vi "Hydrostat.vi"() -> ()   [LabVIEW 2016]
uses:
  <vilib>/express/express signal manip/GetorSetDDTAttributes/Shared VIs/TimeType.ctl
  <vilib>/Waveform/WDTOps.llb/WDT Append Waveforms DBL.vi
  <vilib>/express/express signal manip/GetorSetDDTAttributes/Shared VIs/TimeMode Enum to Boolean.vi
  <vilib>/express/express shared/transition.llb/Dynamic To Waveform Array.vi
  <vilib>/express/express signal manip/GetorSetDDTAttributes/Set DDT Attributes/SetT0.vi
  <vilib>/express/express signal manip/GetorSetDDTAttributes/Set DDT Attributes/sub Set StartTimeStamp.vi
  <vilib>/express/express shared/transition.llb/Waveform Array To Dynamic.vi
  <vilib>/express/express signal manip/GetorSetDDTAttributes/Set DDT Attributes/Set DDT Properties.xnode
  <vilib>/express/express signal manip/GetorSetDDTAttributes/Shared VIs/GetSetShared.lvlib
  <vilib>/express/express signal manip/GetorSetDDTAttributes/Set DDT Attributes/Set DDT Attributes.lvlib
panel:
  in  "Test Name":string caption="Comment"
  in  "Stop Button":bool
  out "Waveform Chart":waveform(dbl)(graph)
  out "PSIA":dbl format="%.2f"
  in  "Outlet":bool
  in  "Mix 2":bool
  in  "Mix 1":bool
  in  "Grease":bool
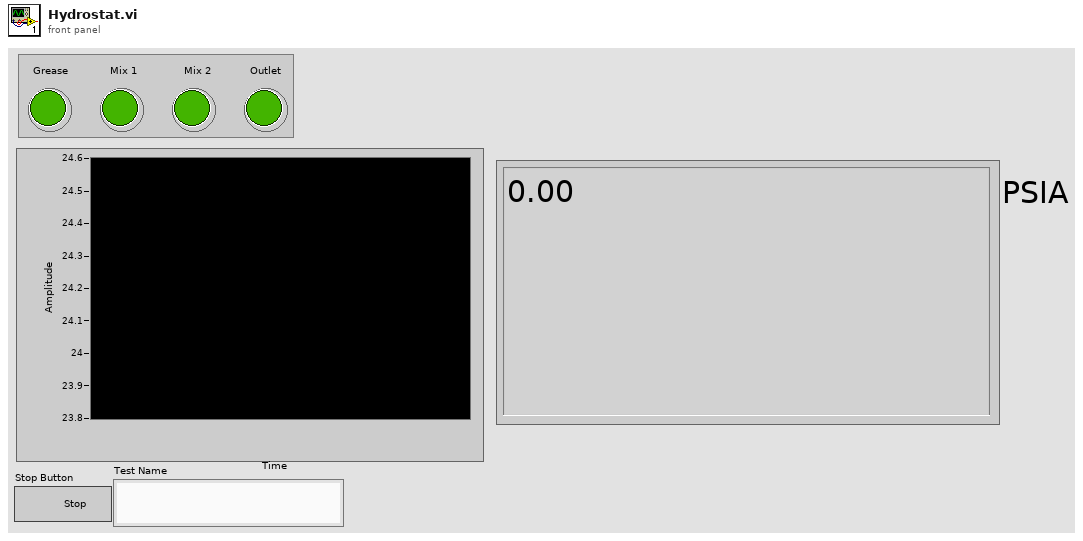
[diagram p1: front panel]
types:
  T1 = typedef "GetSetShared.lvlib/TimeType.ctl" = enum16{"Absolute", "Relative"}
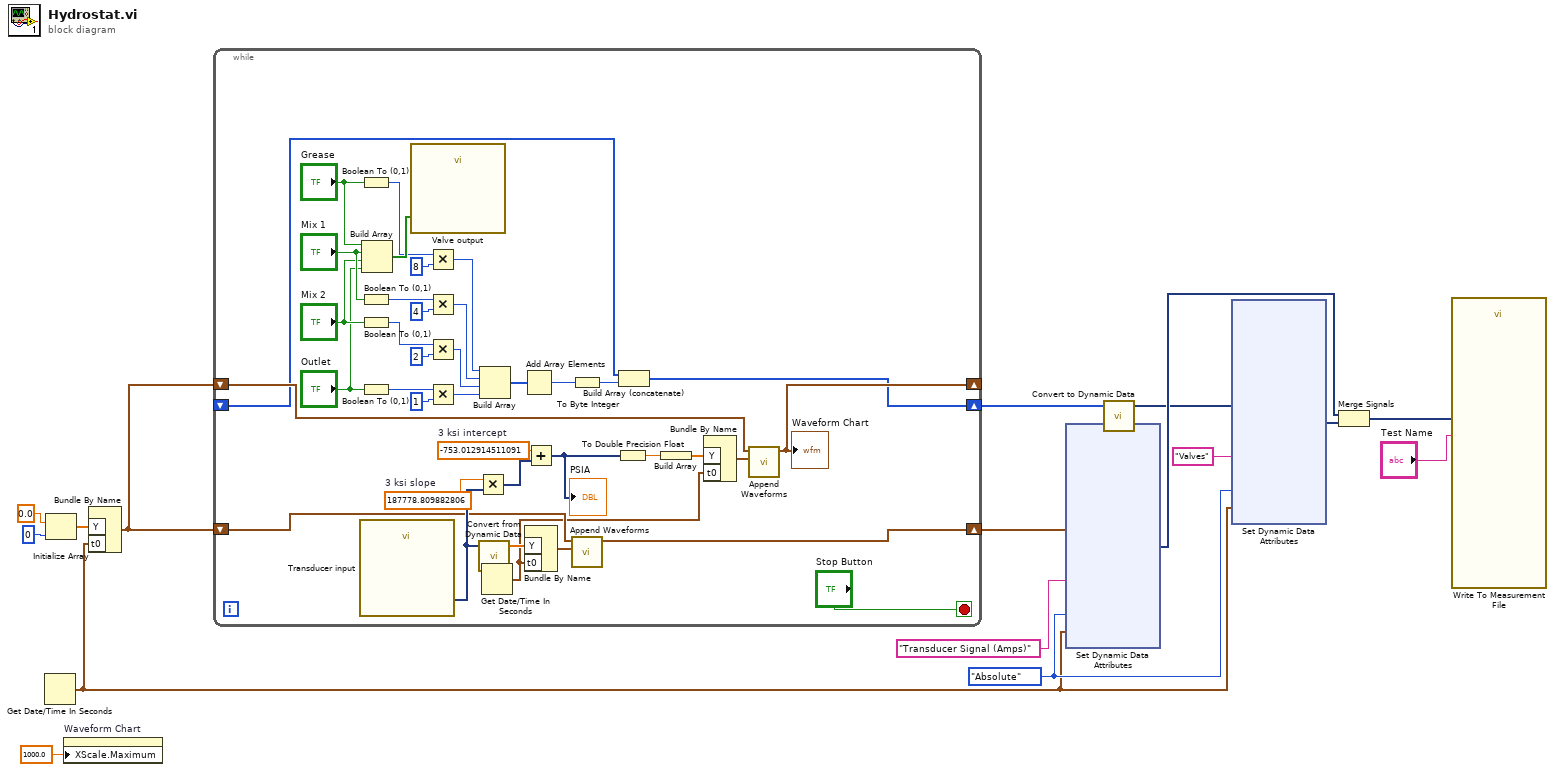
[diagram p0: block diagram]
diagram:
  w4 = TimeType."Absolute" ("Time Mode")
  n1 = Get Date/Time In Seconds() -> (seconds since 1Jan1904=w2:timestamp)
  n2 = Initialize Array(0.0 ("element"), 0 ("dimension size")) -> (w16:dbl[])
  n3 = property on="Waveform Chart" class="WFChart (strict)"("XScale.Maximum"=1000.0 ("Plot Width (samples)")) -> ()  [unwired: 2 in, 2 out]
  n4 = Bundle By Name("Y"=w16, "t0"=w2) -> (w11:waveform(dbl))  [unwired: 1 in]
  n5 = while {
    shift-right: [w49] -> _
    shift-left: w11 -> [w50]
    shift-right: [w38] -> w6
    shift-left: w11 -> [w41]
    shift-right: [w36] -> w3
    shift-left: _ -> [w37]
    stop <- "Stop Button" stop-if-true
    w53 = -753.012914511091  # 3 ksi intercept
    w54 = 187778.809882806  # 3 ksi slope
    n6 = call "Transducer input"() -> ("data"=w44:dynamicdata)  [unwired: 17 in, 2 out]
    n7 = Boolean To (0,1)(Boolean="Grease") -> (0, 1=w24:i16)
    n8 = Boolean To (0,1)(Boolean="Mix 1") -> (0, 1=w25:i16)
    n9 = Boolean To (0,1)(Boolean="Mix 2") -> (0, 1=w26:i16)
    n10 = Boolean To (0,1)(Boolean="Outlet") -> (0, 1=w27:i16)
    n11 = Build Array("Grease", "Mix 1", "Mix 2", "Outlet") -> (w40:bool[])
    n12 = call "Valve output"("data"=w40) -> ()  [unwired: 17 in, 2 out]
    n13 = Multiply(x=w24, y=i16 8) -> (x*y=w31:i16)
    n14 = Multiply(x=w25, y=i16 4) -> (x*y=w30:i16)
    n15 = Multiply(x=w26, y=i16 2) -> (x*y=w29:i16)
    n16 = Multiply(x=w27, y=i16 1) -> (x*y=w28:i16)
    n17 = Multiply(x=w54, y=w44) -> (x*y=w52:dynamicdata)
    n18 = call "Convert from Dynamic Data"("Dynamic Data Type"=w44) -> ("Array"=w43:dbl[])  [unwired: 3 in]
    n19 = Build Array(w31, w30, w29, w28) -> (w19:i16[])
    n20 = Get Date/Time In Seconds() -> (seconds since 1Jan1904=w39:timestamp)
    n21 = Add Array Elements(numeric array=w19) -> (sum=w18:i16)
    n22 = Bundle By Name("Y"=w43, "t0"=w39) -> (w42:waveform(dbl))  [unwired: 1 in]
    n23 = Add(x=w53, y=w52) -> (x+y=w47:dynamicdata)
    "PSIA" <- w47
    n24 = To Byte Integer(number=w18) -> (8bit integer=w17:i8)
    n25 = call-poly <vilib>:"Append Waveforms.vi"("waveform B"=w42, "waveform A"=w41) -> ("waveform out"=w38:waveform(dbl))  [unwired: 8 in, 1 out]
    n26 = To Double Precision Float(number=w47) -> (double precision float=w46:dbl)
    n27 = Build Array (concatenate)(w37, w17) -> (w36:i8[])
    n28 = Build Array(w46) -> (w48:dbl[])
    n29 = Bundle By Name("Y"=w48, "t0"=w39) -> (w45:waveform(dbl))  [unwired: 1 in]
    n30 = call-poly <vilib>:"Append Waveforms.vi"("waveform B"=w45, "waveform A"=w50) -> ("waveform out"=w49:waveform(dbl))  [unwired: 8 in, 1 out]
    "Waveform Chart" <- w49
  }
  n31 = xnode "Set Dynamic Data Attributes"("Signals In"=w6, "Signal Name"="Transducer Signal (Amps)", "Time Mode"=w4, "Start Timestamp"=w2) -> ("Signals Out"=w7:dynamicdata)  [unwired: 3 in, 1 out]
  n32 = call "Convert to Dynamic Data"("Array"=w3) -> ("Dynamic Data Type"=w1:dynamicdata)  [unwired: 3 in]
  n33 = xnode "Set Dynamic Data Attributes"("Signals In"=w1, "Signal Name"="Valves", "Time Mode"=w4, "Start Timestamp"=w2) -> ("Signals Out"=w8:dynamicdata)  [unwired: 3 in, 1 out]
  n34 = Merge Signals(w7, w8) -> (w5:dynamicdata)
  n35 = call "Write To Measurement File"("Signals"=w5, "Comment"="Test Name") -> ()  [unwired: 15 in, 3 out]
